vi "Serialize - Text.vi"(8 "error in":errorcluster, 11 "PPT Data in":refnum<class "PPT Data.lvclass">) -> (0 "error out":errorcluster, 2 "Serialized Text":string, 3 "PPT Data out":refnum<class "PPT Data.lvclass">)   [LabVIEW 2014, in "PPT Library.lvlib" / "PPT Data.lvclass"]
uses:
  PPT Data.lvclass
  PPT Data.lvclass/PPT Data.ctl
  Read P.vi
  Read T.vi
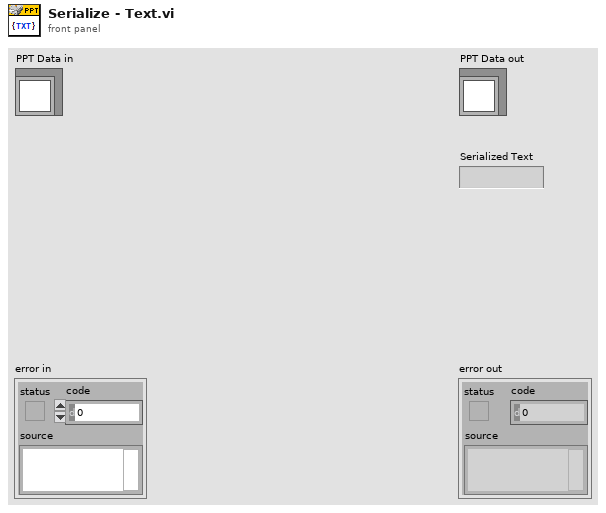
[diagram p1: front panel]
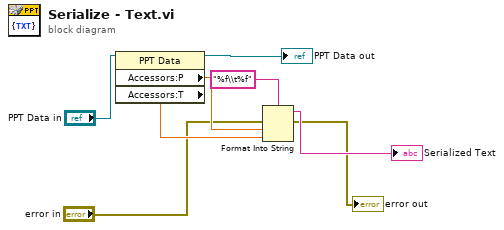
[diagram p0: block diagram]
diagram:
  n1 = property class="PPT Data"(reference="PPT Data in") -> (reference out=→"PPT Data out":refnum<class "PPT Data.lvclass">, "Accessors:P"=w5:dbl, "Accessors:T"=w4:dbl)  [unwired: 1 in, 1 out]
  n2 = Format Into String(format string="%f\\t%f", error in="error in", w5, w4) -> (resulting string=→"Serialized Text":string, error out=→"error out":errorcluster)  [unwired: 1 in]
